vi "New.vi"(7 "Parent":refnum<class "Abstract.lvclass">, 8 "Error In":errorcluster, 11 "Content":string) -> (0 "Error Out":errorcluster, 3 "Text":refnum<class "Text.lvclass">)   [LabVIEW 2018, in "Toolkit.lvlib" / "Nodes.lvlib" / "Text.lvclass"]
uses:
  Text.lvclass
  Abstract/Abstract.lvclass
  Text.lvclass/Text.ctl
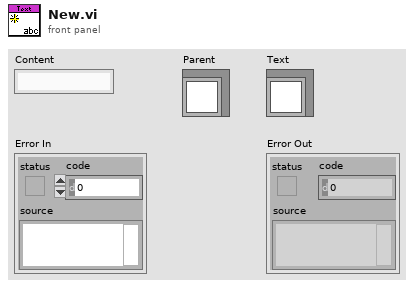
[diagram p1: front panel]
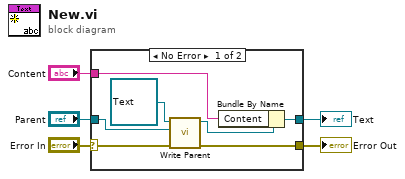
[diagram p0: block diagram]
diagram:
  n1 = case shown="No Error" "Error In" {
    selector: "Error In" -> [w6 w13]
    tunnel: "Parent" -> [w11 _]
    tunnel: [w10 w13] -> w4
    tunnel: "Content" -> [w8 _]
    tunnel: [w7 _] -> w2
    frame No Error {
      n2 = call-dynamic "Write Parent.vi"("Error In"=w6, "Parent"=w11, "Node In"=refnum<class "Text.lvclass"> refnum ("Toolkit.lvlib:Nodes.lvlib:Text.lvclass")) -> ("Error Out"=w10:errorcluster, "Node Out"=w9:refnum<class "Text.lvclass">)  [unwired: 7 in]
      n3 = Bundle By Name(cluster=w9, "Content"=w8) -> (w7:refnum<class "Text.lvclass">)
    }
    frame Error {
    }
  }
  "Text" <- w2
  "Error Out" <- w4
